vi "Command_radio_buttons.vi"(9 "Command Radio Buttons":T1(radio)) -> ()   [LabVIEW 2022 SP3]
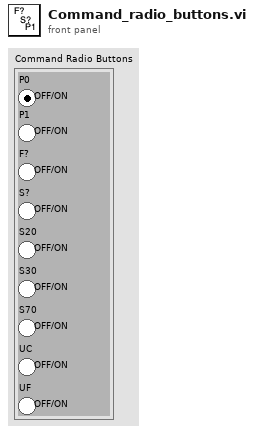
[diagram p1: front panel]
types:
  T1 = enum32{"P0", "P1", "F?", "S?", "S20", "S30", "S70", "UC", "UF"}
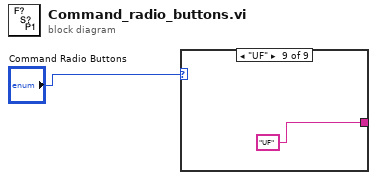
[diagram p0: block diagram]
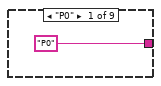
[diagram p2: hidden frame]
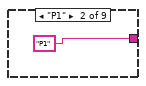
[diagram p3: hidden frame]
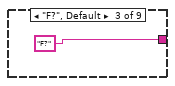
[diagram p4: hidden frame]
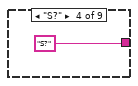
[diagram p5: hidden frame]
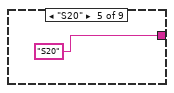
[diagram p6: hidden frame]
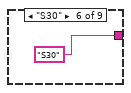
[diagram p7: hidden frame]
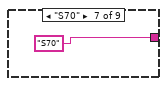
[diagram p8: hidden frame]
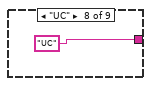
[diagram p9: hidden frame]
diagram:
  n1 = case shown="\"UF\"" "Command Radio Buttons" {
    tunnel: ["P0" "P1" "F?" "S?" "S20" "S30" "S70" "UC" "UF"] -> _
    frame "P0" {
    }
    frame "P1" {
    }
    frame "F?", Default {
    }
    frame "S?" {
    }
    frame "S20" {
    }
    frame "S30" {
    }
    frame "S70" {
    }
    frame "UC" {
    }
    frame "UF" {
    }
  }
